vi "CLD 15 Text String Parsing Solution.vi"(8 "Error In":errorcluster) -> (0 "Error Out":errorcluster)   [LabVIEW 2009]
doc: "CLD 15 This VI reads the file and uses two sub-VI's to parse and then format the file data for use."
uses:
  CLD 15 CSV file data structure.ctl
  <vilib>/Utility/file.llb/Read From Spreadsheet File (string).vi
  <vilib>/Utility/file.llb/Write To Spreadsheet File (string).vi
panel:
  out "File Data":string[][](array[string])
  out "Data Saved to File":string[][](array[string])
  out "Processed Data":T1[](array[typedef])
  # "Processed Data"
  # "Input Data"
  # "Output Data"
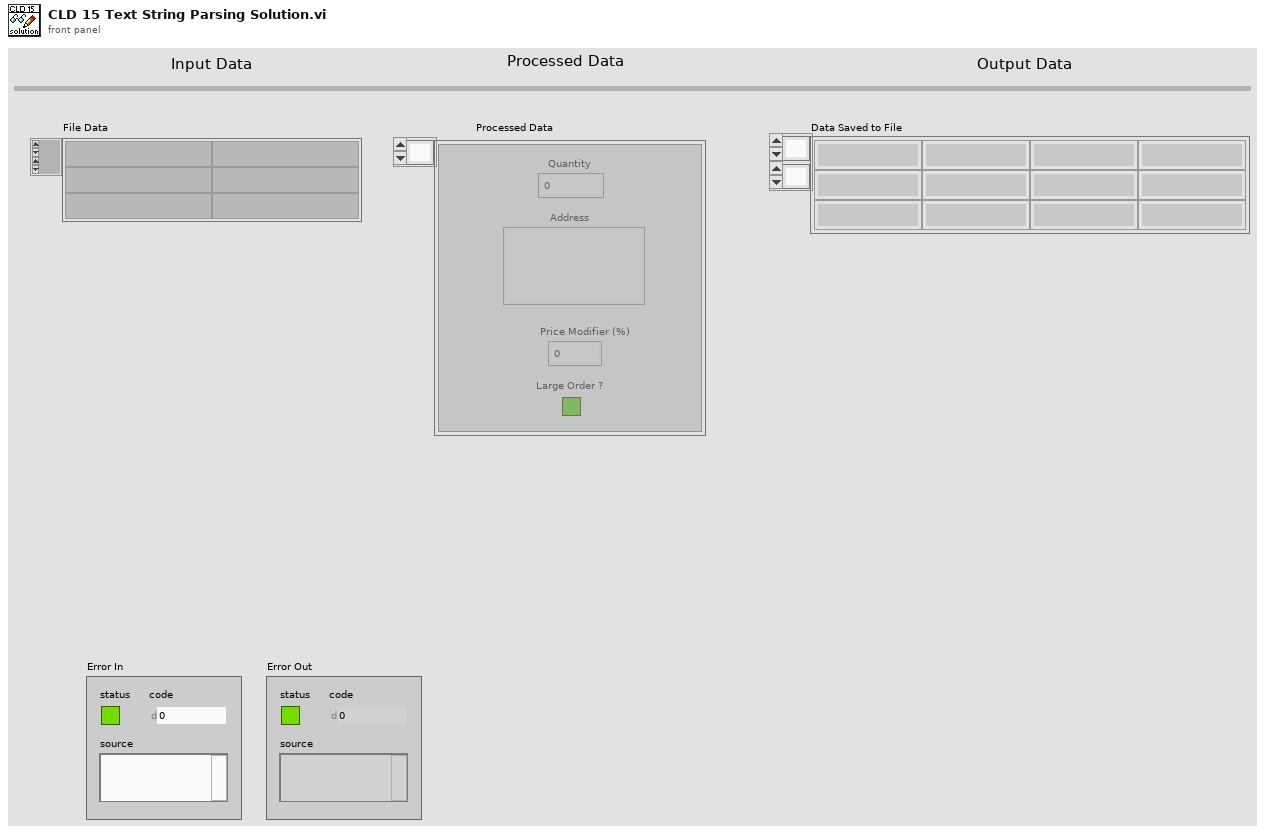
[diagram p1: front panel]
types:
  T1 = typedef "CLD 15 CSV file data structure.ctl" = cluster{"Quantity":i32, "Address":string, "Price Modifier (%)":dbl, "Large Order ?":bool}
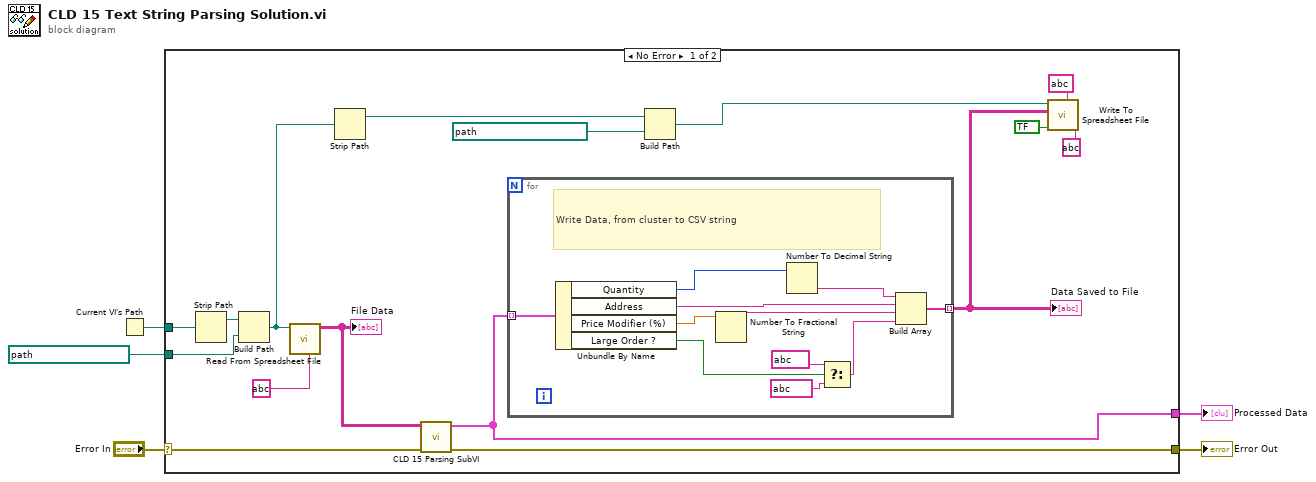
[diagram p0: block diagram]
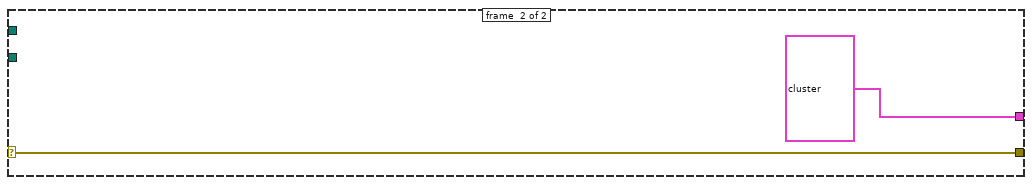
[diagram p2: hidden frame]
diagram:
  n1 = Current VI's Path() -> (path=w4:path)
  n2 = case shown="No Error" "Error In" {
    selector: "Error In" -> [w19 w34]
    tunnel: [w7 T1[] ? ("[Data In]")] -> w1
    tunnel: path ? -> [w21 _]
    tunnel: w4 -> [w20 _]
    tunnel: [w18 w34] -> w2
    frame #0 {
      n3 = Strip Path(path=w20) -> (stripped path=w17:path)  [unwired: 1 out]
      n4 = Build Path(base path=w17, name or relative path=w21) -> (appended path=w6:path)
      n5 = call-poly <vilib>:"Read From Spreadsheet File.vi"("delimiter (\\t)"=string ? ("delimiter (\\t)"), "file path (dialog if empty)"=w6) -> ("all rows"=w16:string[][])  [unwired: 5 in, 4 out]
      "File Data" <- w16
      n6 = Strip Path(path=w6) -> (stripped path=w11:path)  [unwired: 1 out]
      n7 = call "CLD 15 Parsing SubVI.vi"("Error In"=w19, "all rows in"=w16) -> ("Error Out"=w18:errorcluster, "Data Out"=w7:T1[])  [unwired: 8 in]
      n8 = for {
        tunnel: w7 -> [w32] mode=indexing
        tunnel: [w23] -> w14 mode=indexing
        # "Write Data, from cluster to CSV string"
        n9 = Unbundle By Name(w32) -> ("Quantity"=w31:i32, "Address"=w25:string, "Price Modifier (%)"=w30:dbl, "Large Order ?"=w29:bool)
        n10 = Number To Fractional String(number=w30) -> (F-format string=w24:string)  [unwired: 3 in]
        n11 = Number To Decimal String(number=w31) -> (decimal integer string=w26:string)  [unwired: 1 in]
        n12 = Select(t=string ?, s=w29, f=string ?) -> (s? t:f=w22:string)
        n13 = Build Array(w26, w25, w24, w22) -> (w23:string[])
      }
      "Data Saved to File" <- w14
      n14 = Build Path(base path=w11, name or relative path=path ?) -> (appended path=w9:path)
      n15 = call-poly <vilib>:"Write To Spreadsheet File.vi"("delimiter (\\t)"=string ? ("delimiter (\\t)"), "format (%s)"=string ?, "append to file? (new file:F)"=bool ?, "2D data"=w14, "file path (dialog if empty)"=w9) -> ()  [unwired: 3 in, 1 out]
    }
    frame #1 {
    }
  }
  "Error Out" <- w2
  "Processed Data" <- w1
